vi "Parse Identifier List.vi"(11 "string":string) -> (3 "identifier list":string[](array[string]))   [LabVIEW 2024, in "Logging.lvlib" / "Format String.lvclass"]
uses:
  Format String.lvclass
panel:
  # "Connector Pane"
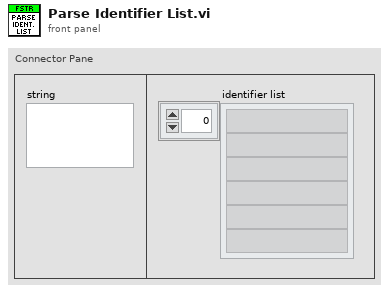
[diagram p1: front panel]
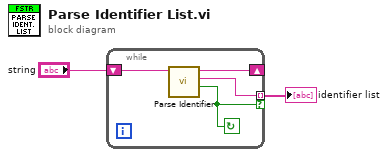
[diagram p0: block diagram]
diagram:
  n1 = while {
    shift-right: [w5] -> _
    shift-left: "string" -> [w6]
    tunnel: [w4] -> w2 mode=indexing if=w3
    stop <- w3 continue-if-true
    n2 = call "Parse Identifier.vi"("string"=w6) -> ("found?"=w3:bool, "identifier"=w4:string, "remaining string"=w5:string)  [unwired: 8 in]
  }
  "identifier list" <- w2
